vi "loadBoard.vi"(8 "error in (no error)":errorcluster, 11 "CQT_DDS in":refnum<class "CQT_DDS.lvclass">) -> (0 "error out":errorcluster, 3 "CQT_DDS out":refnum<class "CQT_DDS.lvclass">)   [LabVIEW 2009, in "Hardware.lvlib" / "Channels.lvlib" / "CQT_DDS.lvclass"]
uses:
  CQT_DDS.lvclass
  CQT_DDS.lvclass/CQT_DDS.ctl
  C:/Program Files/National Instruments/LabVIEW 2009/instr.lib/CQT_DDS/DDSLibrary/20111109/CQTAD9958.dll
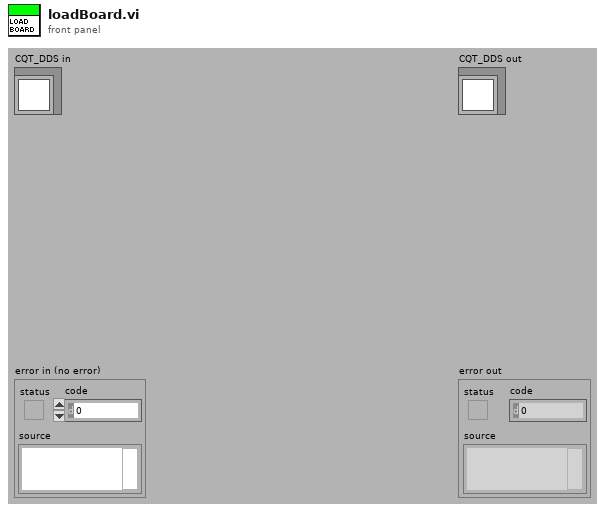
[diagram p1: front panel]
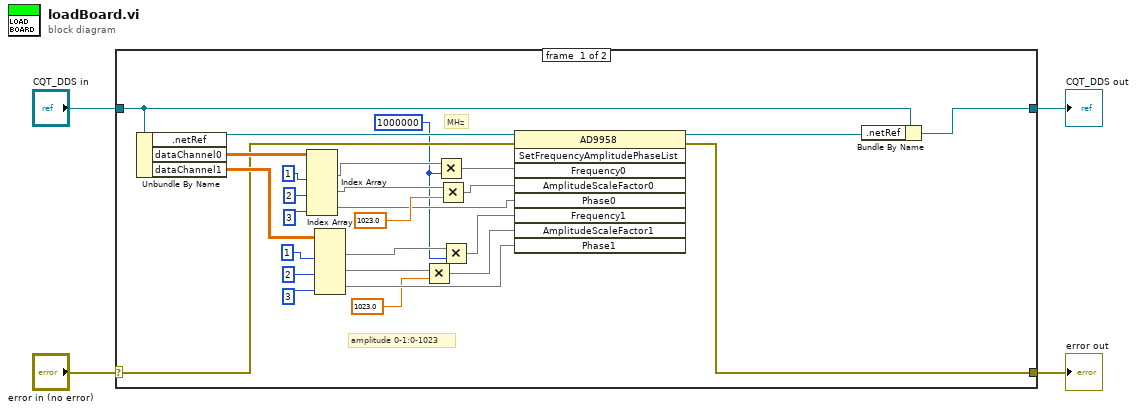
[diagram p0: block diagram]
diagram:
  n1 = case shown="No Error" "error in (no error)" {
    selector: "error in (no error)" -> [w22 w33]
    tunnel: [w15 w33] -> w3
    tunnel: [w20 w32] -> w1
    tunnel: "CQT_DDS in" -> [w21 w32]
    frame #0 {
      w5 = 1000000
      # "amplitude 0-1:0-1023"
      # "MHz"
      n2 = Unbundle By Name(w21) -> (".netRef"=w23:refnum<k24>, "dataChannel0"=w31:dbl[][], "dataChannel1"=w24:dbl[][])
      n3 = Index Array(array=w31, index (col) #1=1, index (col) #2=2, index (col) #3=3) -> (element #1=w19:dbl[], element #2=w13:dbl[], element #3=w8:dbl[])  [unwired: 3 in]
      n4 = Index Array(array=w24, index (col) #1=1, index (col) #2=2, index (col) #3=3) -> (element #1=w18:dbl[], element #2=w11:dbl[], element #3=w17:dbl[])  [unwired: 3 in]
      n5 = Multiply(x=w11, y=1023.0) -> (x*y=w10:dbl[])
      n6 = Multiply(x=w19, y=w5) -> (x*y=w9:dbl[])
      n7 = Multiply(x=w13, y=1023.0) -> (x*y=w7:dbl[])
      n8 = Multiply(x=w18, y=w5) -> (x*y=w6:dbl[])
      n9 = invoke class="AD9958" method="SetFrequencyAmplitudePhaseList"(reference=w23, error in=w22, "Frequency0"=w9, "AmplitudeScaleFactor0"=w7, "Phase0"=w8, "Frequency1"=w6, "AmplitudeScaleFactor1"=w10, "Phase1"=w17) -> (reference out=w16:refnum<k24>, error out=w15:errorcluster)  [unwired: 1 in, 7 out]
      n10 = Bundle By Name(cluster=w21, ".netRef"=w16) -> (w20:refnum<class "CQT_DDS.lvclass">)
    }
    frame #1 {
    }
  }
  "error out" <- w3
  "CQT_DDS out" <- w1
